vi "Line Detector Process.vi"(8 "error in (no error)":errorcluster, 9 "Best fit guess":dbl[][](array[numeric]) format="%#_4p", 10 "File":path=path "C:/Data/April_2017/042017/ru112_042017.tdms", 11 "Line Detector Configuration":T1={"Peak width guess"=500.0, "Background removal"=enum."High-pass", "Smoothing"=enum."Low-pass", "Smooth window"=200.0, "Relative threshold"=0.2, "Finder algorithm"=enum."Wavelet", "Bgd window"=50000.0, "Spectrum recorder module name"="Spectrum Recorder", "Fit window"=1000.0, "Initial fit guess"=enum."Peak finder", "...with header "="", "Follow\npeaks"=FALSE, "Re-sample"=nan, "rusin\n.dat"=enum."NONE"} {"Re-sample" format="%#_6pHz"; "Fit window" format="%#_6pHz"; "Bgd window" format="%#_6pHz"; "Smooth window" format="%#_6pHz"; "Peak width guess" format="%#_6pHz"}) -> (0 "error out":errorcluster, 1 "Plots":cluster{"X":dbl[], "Array":dbl[]}[](array[cluster]), 2 "File out":path, 3 "Best fit results":dbl[][](array[numeric]) format="%#_4p", 4 "Peak Plot":cluster{"Ramp Pattern":dbl[], "X":dbl[]}[](graph), 5 "Peaks":dbl[](array[numeric]) format="%#_4p", 6 "sp time":timestamp)   [LabVIEW 2016]
uses:
  LabActor/Post-Processors/Line Detector/Line Detector Configuration.ctl
panel:
  # "F0         dF     Ampl   Phase   Xbgrd   Ybgrd"
  # "F0         dF     Ampl   Phase   Xbgrd   Ybgrd"
  # "Peak finder config"
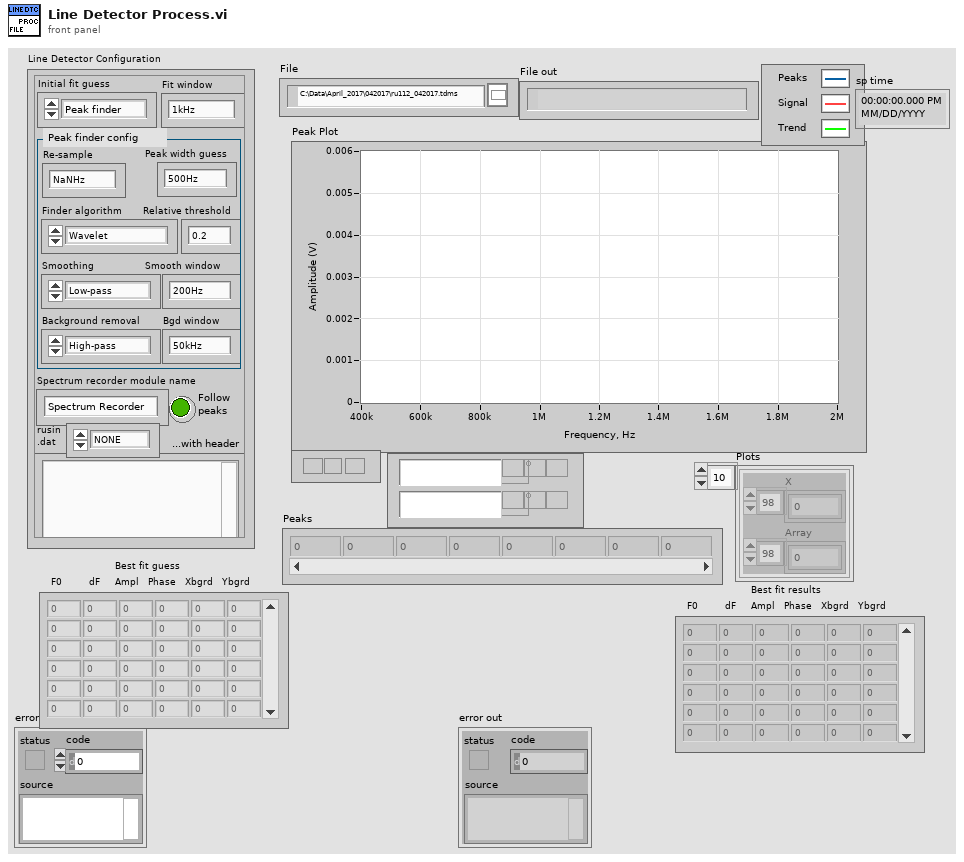
[diagram p1: front panel]
types:
  T1 = typedef "Line Detector Configuration.ctl" = cluster{"Peak width guess":dbl, "Background removal":enum16{"NONE", "High-pass", "Detrend"}, "Smoothing":enum16{"NONE", "Low-pass", "Denoise"}, "Smooth window":dbl, "Relative threshold":dbl, "Finder algorithm":enum16{"Basic", "Wavelet", "Wavelet+detrend"}, "Bgd window":dbl, "Spectrum recorder module name":string, "Fit window":dbl, "Initial fit guess":enum16{"Peak finder", "Last fit"}, "...with header ":string, "Follow\npeaks":bool, "Re-sample":dbl, "rusin\n.dat":enum16{"NONE", "DINES/cm2", "GPa"}}
  T2 = typedef "Spectrum Configuration.ctl" = cluster{"Start frequency":dbl, "End frequency":dbl, "Frequency step":dbl, "Step duration":dbl, "Red Pitaya address":string, "Open plot \non start":bool, "Focus region centers":dbl[], "Regions width":dbl, "Out-of-focus\nstep acceleration":i32}
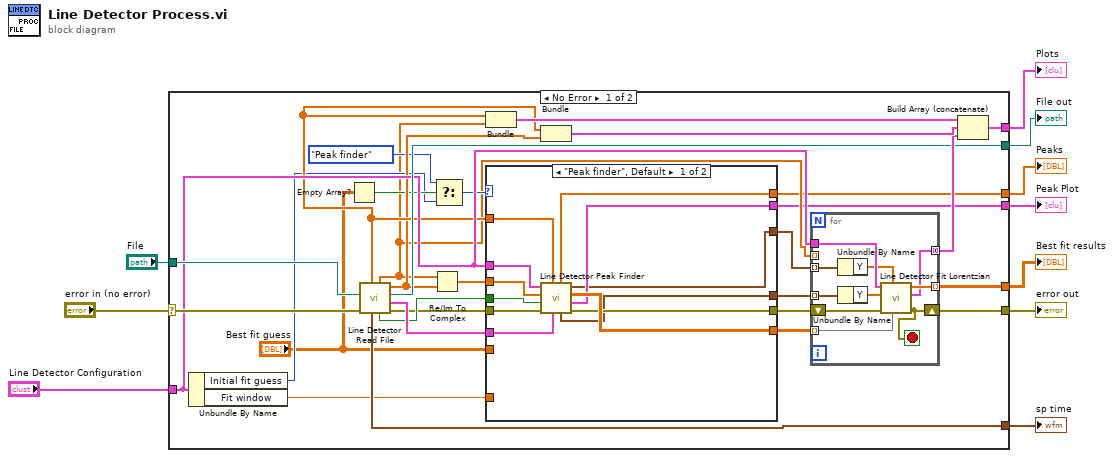
[diagram p0: block diagram]
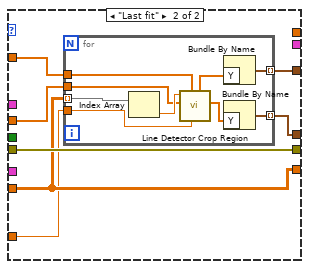
[diagram p2: hidden frame]
diagram:
  n1 = case shown="No Error" "error in (no error)" {
    selector: "error in (no error)" -> [w34 w79]
    tunnel: "File" -> [w36 w80]
    tunnel: [w33 w80] -> w8
    tunnel: "Line Detector Configuration" -> [w30 _]
    tunnel: [w31 w79] -> w6
    tunnel: [w16 _] -> w4
    tunnel: [w32 _] -> w1
    tunnel: [w37 _] -> w5
    tunnel: [w12 _] -> w3
    tunnel: [w35 _] -> w2
    frame No Error {
      n2 = Unbundle By Name(w30) -> ("Initial fit guess"=w22:enum16{"Peak finder", "Last fit"}, "Fit window"=w13:dbl)
      n3 = Empty Array?(array="Best fit guess") -> (empty?=w24:bool)
      n4 = call "Line Detector Read File.vi"("error in (no error)"=w34, "File"=w36) -> ("error out"=w15:errorcluster, "Spectrum Recorder Configuration"=w28:T2, "File out"=w33:path, "Signal Y"=w25:dbl[], "found?"=w27:bool, "Signal X"=w19:dbl[], "sp time"=w35:timestamp, "Frequency"=w29:dbl[])  [unwired: 2 in]
      n5 = Re/Im To Complex(1:w25, 2:w19) -> (0:w26:cdb[])
      n6 = Select(t=enum16{"Peak finder", "Last fit"}."Peak finder" ("Initial fit guess"), s=w24, f=w22) -> (s? t:f=w21:enum16{"Peak finder", "Last fit"})
      n7 = Bundle("Frequency"=w29, "Signal X"=w19) -> (w40:cluster{"Frequency":dbl[], "Signal X":dbl[]})  [unwired: 1 in]
      n8 = case shown="\"Peak finder\", Default" w21 {
        tunnel: w30 -> [w52 _]
        tunnel: w29 -> [w51 w57]
        tunnel: w28 -> [w50 _]
        tunnel: w27 -> [w43 _]
        tunnel: w26 -> [w49 w56]
        tunnel: w15 -> [w48 w59]
        tunnel: [w47 w58] -> w17
        tunnel: "Best fit guess" -> [_ w58]
        tunnel: [w46 _] -> w16
        tunnel: [w45 w59] -> w14
        tunnel: [w44 _] -> w12
        tunnel: [w42 w53] -> w20
        tunnel: [w41 w54] -> w18
        tunnel: w13 -> [_ w55]
        frame "Peak finder", Default {
          n9 = call "Line Detector Peak Finder.vi"("Spectrum Recorder Configuration"=w50, "Frequency"=w51, "error in (no error)"=w48, "Valid Spectrum Recorder Configuration"=w43, "Signal"=w49, "Line Detector Configuration"=w52) -> ("error out"=w45:errorcluster, "Peak Plot"=w46:cluster{"Ramp Pattern":dbl[], "X":dbl[]}[], "Initial fit guess"=w47:dbl[][], "Regions frequencies"=w42:waveform(dbl)[], "Regions signals"=w41:waveform(cdb)[], "Peaks"=w44:dbl[])
        }
        frame "Last fit" {
          n10 = for {
            tunnel: w58 -> [w68] mode=indexing
            tunnel: w57 -> [w64]
            tunnel: w56 -> [w66]
            tunnel: w55 -> [w65]
            tunnel: [w62] -> w54 mode=indexing
            tunnel: [w61] -> w53 mode=indexing
            n11 = Index Array(array=w68) -> (element=w67:dbl)  [unwired: 1 in]
            n12 = call "Line Detector Crop Region.vi"("Region width"=w65, "Frequency"=w64, "Signal"=w66, "Center frequency"=w67) -> ("Signal  out"=w63:cdb[], "Frequency out"=w60:dbl[])  [unwired: 4 in, 2 out]
            n13 = Bundle By Name("Y"=w60) -> (w61:waveform(dbl))  [unwired: 1 in]
            n14 = Bundle By Name("Y"=w63) -> (w62:waveform(cdb))  [unwired: 1 in]
          }
        }
      }
      n15 = Bundle("Frequency"=w29, "Signal Y"=w25) -> (w39:cluster{"Frequency":dbl[], "Signal Y":dbl[]})  [unwired: 1 in]
      n16 = for {
        tunnel: w30 -> [w78]
        shift-right: [w69] -> w31
        shift-left: w14 -> [w75]
        tunnel: [w77] -> w32 mode=indexing
        tunnel: [w76] -> w38 mode=concatenating
        tunnel: w20 -> [w72] mode=indexing
        tunnel: w19 -> [_] mode=indexing
        tunnel: w18 -> [w74] mode=indexing
        tunnel: w17 -> [w73] mode=indexing
        stop <- w69 stop-if-true
        n17 = Unbundle By Name(w72) -> ("Y"=w71:dbl[])
        n18 = Unbundle By Name(w74) -> ("Y"=w70:cdb[])
        n19 = call "Line Detector Fit Lorentzian.vi"("Guess"=w73, "Frequency"=w71, "Error In"=w75, "Signal"=w70, "Line Detector Configuration"=w78) -> ("Error Out"=w69:errorcluster, "Plot"=w76:cluster{"X":dbl[], "Array":dbl[]}[], "best fit parameters"=w77:dbl[])  [unwired: 4 in]
      }
      n20 = Build Array (concatenate)(w40, w39, w38) -> (w37:cluster{"X":dbl[], "Array":dbl[]}[])
    }
    frame Error {
    }
  }
  "error out" <- w6
  "File out" <- w8
  "Plots" <- w5
  "Peak Plot" <- w4
  "Peaks" <- w3
  "sp time" <- w2
  "Best fit results" <- w1
